vi "FGV - DO.vi"(8 "error in":errorcluster, 10 "Digital Outs":bool[](array[boolean])=[FALSE, FALSE, FALSE, FALSE], 11 "State":T1) -> (0 "error out":errorcluster, 2 "Digital Out":bool[](array[boolean]))   [LabVIEW 2017]
doc: "v1.1:\n- 2WR motor selection\n\nv1.0:\n- VI Created"
uses:
  controls/FGV DO.ctl
  <vilib>/DAQmx/write.llb/DAQmx Write (Digital 1D Bool NChan 1Samp 1Line).vi
  <vilib>/DAQmx/miscellaneous.llb/DAQmx Fill In Error Info.vi
panel:
  in  "Digital Out 2":bool[](array[boolean])=[FALSE, FALSE, FALSE, FALSE, FALSE, FALSE, FALSE, FALSE, FALSE, FALSE, FALSE]
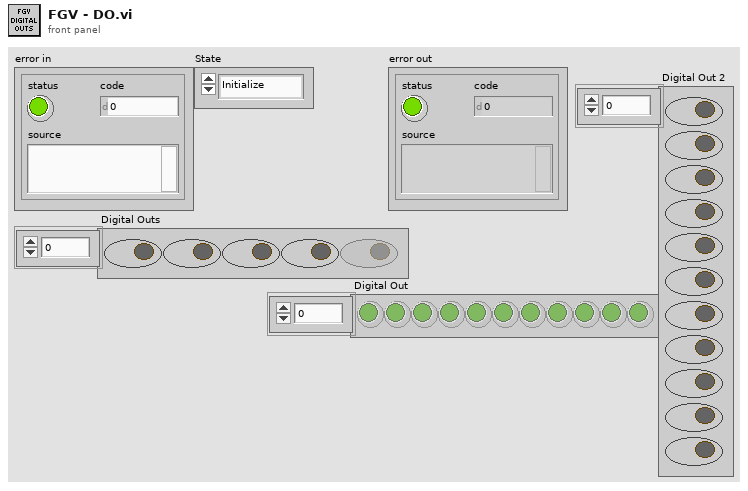
[diagram p1: front panel]
types:
  T1 = typedef "FGV DO.ctl" = enum16{"Initialize", "Start Task", "Clamping", "Load CYL", "Contactors", "Loadcell CYL", "BSL", "Read DO", "Clear Tasks", "Clear Task"}
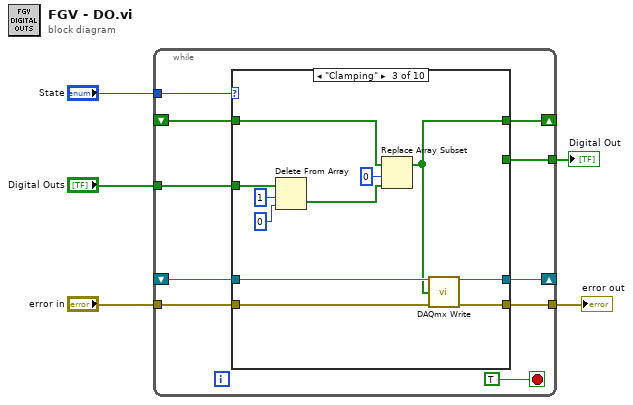
[diagram p0: block diagram]
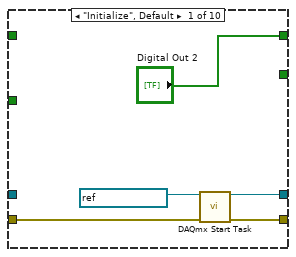
[diagram p2: hidden frame]
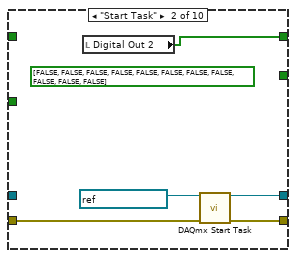
[diagram p3: hidden frame]
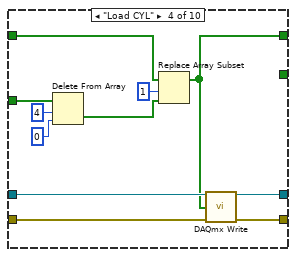
[diagram p4: hidden frame]
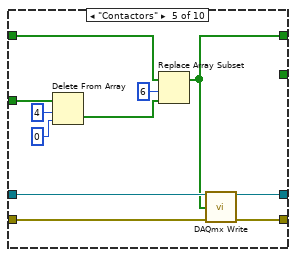
[diagram p5: hidden frame]
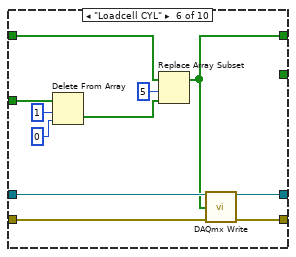
[diagram p6: hidden frame]
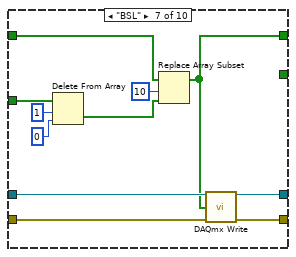
[diagram p7: hidden frame]
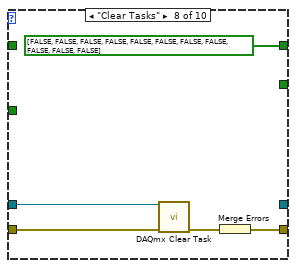
[diagram p8: hidden frame]
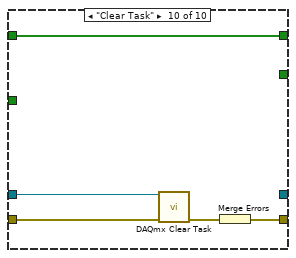
[diagram p10: hidden frame]
diagram:
  n1 = while {
    shift-right: [w14] -> _
    shift-left: _ -> [w9]
    tunnel: "State" -> [w15]
    shift-right: [w13] -> _
    shift-left: _ -> [w10]
    tunnel: "error in" -> [w11]
    tunnel: [w12] -> w3
    tunnel: "Digital Outs" -> [w8]
    tunnel: [w6] -> w1
    stop <- TRUE stop-if-true
    n2 = case shown="\"Clamping\"" w15 {
      tunnel: ["Digital Out 2" w21 w30 w41 w52 w63 w74 bool[] [FALSE, FALSE, FALSE, FALSE, FALSE, FALSE, FALSE, FALSE, FALSE, FALSE, FALSE] ("Digital Out") w88 w89] -> w14
      tunnel: [w16 w22 w32 w43 w54 w65 w76 _ w87 _] -> w13
      tunnel: [w17 w23 w35 w46 w57 w68 w79 w84 w86 w93] -> w12
      tunnel: w11 -> [w18 w24 w36 w47 w58 w69 w80 w81 w86 w90]
      tunnel: w10 -> [_ _ w33 w44 w55 w66 w77 w83 w87 w92]
      tunnel: w9 -> [_ _ w31 w42 w53 w64 w75 _ w88 w89]
      tunnel: w8 -> [_ _ w29 w40 w51 w62 w73 _ _ _]
      tunnel: [_ _ _ _ _ _ _ _ w88 _] -> w6
      frame "Initialize", Default {
        n3 = call <vilib>:"DAQmx Start Task.vi"("task/channels in"=refnum<k21> "1922_AllDO", "error in"=w18) -> ("task out"=w16:refnum<k21>, "error out"=w17:errorcluster)  [unwired: 12 in]
      }
      frame "Start Task" {
        (unwired) bool[] [FALSE, FALSE, FALSE, FALSE, FALSE, FALSE, FALSE, FALSE, FALSE, FALSE, FALSE] ("Digital Out")
        n4 = local read "Digital Out 2"() -> (w21:bool[])
        n5 = call <vilib>:"DAQmx Start Task.vi"("task/channels in"=refnum<k21> "1922_AllDO", "error in"=w24) -> ("task out"=w22:refnum<k21>, "error out"=w23:errorcluster)  [unwired: 12 in]
      }
      frame "Clamping" {
        n6 = Delete From Array(array=w29, length=1, index=0) -> (deleted portion=w26:bool[])  [unwired: 1 out]
        n7 = Replace Array Subset(array=w31, new element=w26, index=0) -> (w30:bool[])
        n8 = call-poly <vilib>:"DAQmx Write.vi"("task/channels in"=w33, "data"=w30, "error in"=w36) -> ("task out"=w32:refnum<k21>, "error out"=w35:errorcluster)  [unwired: 10 in, 1 out]
      }
      frame "Load CYL" {
        n9 = Delete From Array(array=w40, length=4, index=0) -> (deleted portion=w37:bool[])  [unwired: 1 out]
        n10 = Replace Array Subset(array=w42, new element=w37, index=1) -> (w41:bool[])
        n11 = call-poly <vilib>:"DAQmx Write.vi"("task/channels in"=w44, "data"=w41, "error in"=w47) -> ("task out"=w43:refnum<k21>, "error out"=w46:errorcluster)  [unwired: 10 in, 1 out]
      }
      frame "Contactors" {
        n12 = Delete From Array(array=w51, length=4, index=0) -> (deleted portion=w48:bool[])  [unwired: 1 out]
        n13 = Replace Array Subset(array=w53, new element=w48, index=6) -> (w52:bool[])
        n14 = call-poly <vilib>:"DAQmx Write.vi"("task/channels in"=w55, "data"=w52, "error in"=w58) -> ("task out"=w54:refnum<k21>, "error out"=w57:errorcluster)  [unwired: 10 in, 1 out]
      }
      frame "Loadcell CYL" {
        n15 = Delete From Array(array=w62, length=1, index=0) -> (deleted portion=w59:bool[])  [unwired: 1 out]
        n16 = Replace Array Subset(array=w64, new element=w59, index=5) -> (w63:bool[])
        n17 = call-poly <vilib>:"DAQmx Write.vi"("task/channels in"=w66, "data"=w63, "error in"=w69) -> ("task out"=w65:refnum<k21>, "error out"=w68:errorcluster)  [unwired: 10 in, 1 out]
      }
      frame "BSL" {
        n18 = Delete From Array(array=w73, length=1, index=0) -> (deleted portion=w70:bool[])  [unwired: 1 out]
        n19 = Replace Array Subset(array=w75, new element=w70, index=10) -> (w74:bool[])
        n20 = call-poly <vilib>:"DAQmx Write.vi"("task/channels in"=w77, "data"=w74, "error in"=w80) -> ("task out"=w76:refnum<k21>, "error out"=w79:errorcluster)  [unwired: 10 in, 1 out]
      }
      frame "Clear Tasks" {
        n21 = call <vilib>:"DAQmx Clear Task.vi"("task in"=w83, "error in"=w81) -> ("error out"=w82:errorcluster)  [unwired: 13 in]
        n22 = Merge Errors(w82) -> (w84:errorcluster)
      }
      frame "Read DO" {
      }
      frame "Clear Task" {
        n23 = call <vilib>:"DAQmx Clear Task.vi"("task in"=w92, "error in"=w90) -> ("error out"=w91:errorcluster)  [unwired: 13 in]
        n24 = Merge Errors(w91) -> (w93:errorcluster)
      }
    }
  }
  "error out" <- w3
  "Digital Out" <- w1
